vi "AlphaBeta.vi"() -> ()   [LabVIEW 2017]
uses:
  AlphaBetaAndDQ_variants/ABCtoAlphaBeta_3PhaseUnitaryMagnitude_src.vi
  AlphaBetaAndDQ_variants/AlphaBetaToABC_UnitaryMagnitude_src.vi
  AlphaBetaAndDQ_variants/ABCtoAlphaBeta_3PhasePowerInvariant_src.vi
  AlphaBetaAndDQ_variants/AlphaBetaToABC_PowerInvariant_src.vi
  AlphaBetaAndDQ_variants/ABCtoAlphaBeta_2PhaseUnitaryMagnitude_src.vi
  AlphaBetaAndDQ_variants/ABCtoAlphaBeta_2PhasePowerInvariant_src.vi
  <vilib>/Analysis/NI_AALBase.lvlib
panel:
  out "transposed array":sgl[][](graph)
  out "3 phase UM error stddev":dbl format="%0.2f"
  out "3 phase PI error stddev":dbl format="%0.2f"
  out "2 phase UM error stddev":dbl format="%0.2f"
  out "2 phase PI error stddev":dbl format="%0.2f"
  in  "Imbalance (percent)":dbl
  in  "GridImbalance":bool
  in  "Noise Magnitude (percent)":dbl
  in  "InjectAdditiveNoise":bool
  out "3 phase UM error mean":dbl format="%0.2f"
  out "3 phase UM error max":dbl
  out "3 phase PI error mean":dbl format="%0.2f"
  out "3 phase PI error max":dbl
  out "2 phase UM error mean":dbl format="%0.2f"
  out "2 phase UM error max":dbl
  in  "Magnitude":dbl=1.0
  out "2 phase PI error max":dbl
  out "2 phase PI error mean":dbl format="%0.2f"
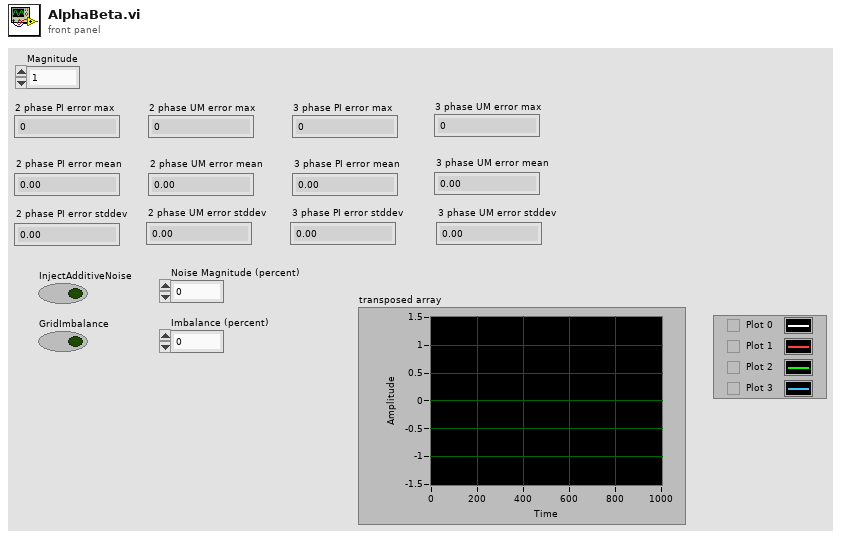
[diagram p1: front panel]
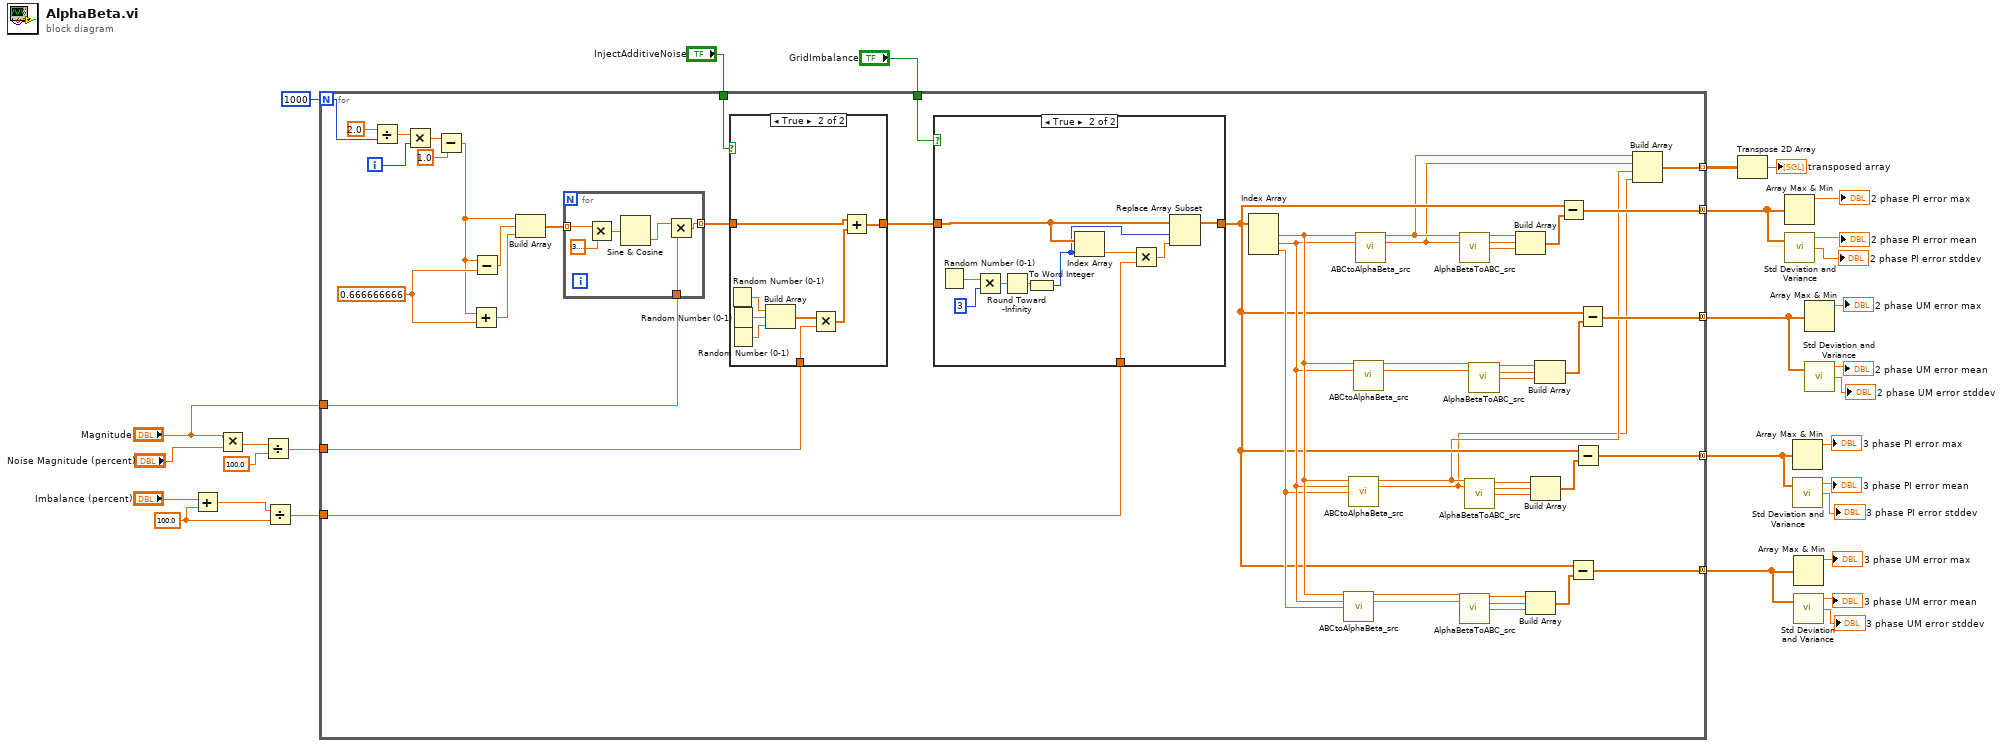
[diagram p0: block diagram]
diagram:
  w8 = 100.0 ("y")
  n1 = Add(x="Imbalance (percent)", y=w8) -> (x+y=w9:dbl)
  n2 = Multiply(x="Magnitude", y="Noise Magnitude (percent)") -> (x*y=w16:dbl)
  n3 = Divide(x=w16, y=100.0) -> (x/y=w13:dbl)
  n4 = Divide(x=w9, y=w8) -> (x/y=w7:dbl)
  n5 = for {
    N: 1000 -> [w47]
    tunnel: [w41] -> w27 mode=concatenating
    tunnel: [w40] -> w24 mode=concatenating
    tunnel: [w39] -> w21 mode=concatenating
    tunnel: [w38] -> w18 mode=concatenating
    tunnel: "Magnitude" -> [w55]
    tunnel: w13 -> [w54]
    tunnel: "InjectAdditiveNoise" -> [w53]
    tunnel: "GridImbalance" -> [w52]
    tunnel: w7 -> [w50]
    tunnel: [w31] -> w2 mode=indexing
    i -> [w45]
    w81 = 0.666666666
    n6 = Divide(x=2.0, y=w47) -> (x/y=w46:dbl)
    n7 = Multiply(x=w46, y=w45) -> (x*y=w44:dbl)
    n8 = Subtract(x=w44, y=1.0) -> (x-y=w42:dbl)
    n9 = Add(x=w42, y=w81) -> (x+y=w79:dbl)
    n10 = Subtract(x=w42, y=w81) -> (x-y=w78:dbl)
    n11 = Build Array(w42, w78, w79) -> (w80:dbl[])
    n12 = for {
      tunnel: w80 -> [w107] mode=indexing
      tunnel: [w104] -> w56 mode=indexing
      tunnel: w55 -> [w103]
      n13 = Multiply(x=w107, y=3.141592653589793) -> (x*y=w105:dbl)
      n14 = Sine & Cosine(0:w105) -> (2:w102:dbl)  [unwired: 1 out]
      n15 = Multiply(x=w102, y=w103) -> (x*y=w104:dbl)
    }
    n16 = case shown="True" w53 {
      tunnel: w56 -> [w93 w95]
      tunnel: [w93 w94] -> w51
      tunnel: w54 -> [_ w97]
      frame False {
      }
      frame True {
        n17 = Random Number (0-1)() -> (number: 0 to 1=w100:dbl)
        n18 = Random Number (0-1)() -> (number: 0 to 1=w101:dbl)
        n19 = Random Number (0-1)() -> (number: 0 to 1=w99:dbl)
        n20 = Build Array(w100, w101, w99) -> (w98:dbl[])
        n21 = Multiply(x=w98, y=w97) -> (x*y=w96:dbl[])
        n22 = Add(x=w95, y=w96) -> (x+y=w94:dbl[])
      }
    }
    n23 = case shown="True" w52 {
      tunnel: w51 -> [w82 w86]
      tunnel: w50 -> [_ w87]
      tunnel: [w82 w84] -> w49
      frame False {
      }
      frame True {
        n24 = Random Number (0-1)() -> (number: 0 to 1=w92:dbl)
        n25 = Multiply(x=w92, y=3) -> (x*y=w90:dbl)
        n26 = Round Toward -Infinity(1:w90) -> (0:w89:dbl)
        n27 = To Word Integer(number=w89) -> (16bit integer=w83:i16)
        n28 = Index Array(array=w86, index=w83) -> (element=w88:dbl)
        n29 = Multiply(x=w88, y=w87) -> (x*y=w85:dbl)
        n30 = Replace Array Subset(array=w86, new element=w85, index=w83) -> (w84:dbl[])
      }
    }
    n31 = Index Array(array=w49) -> (element #1=w59:dbl, element #2=w58:dbl, element #3=w57:dbl)  [unwired: 3 in]
    n32 = call-poly "ABCtoAlphaBeta_src.vi"("A"=w59, "B"=w58, "C"=w57) -> ("alpha"=w60:sgl, "beta"=w61:sgl)  [unwired: 11 in]
    n33 = call-poly "ABCtoAlphaBeta_src.vi"("A"=w59, "B"=w58, "C"=w57) -> ("alpha"=w33:sgl, "beta"=w32:sgl)  [unwired: 11 in]
    n34 = call-poly "ABCtoAlphaBeta_src.vi"("A"=w59, "B"=w58) -> ("alpha"=w37:sgl, "beta"=w36:sgl)  [unwired: 12 in]
    n35 = call-poly "ABCtoAlphaBeta_src.vi"("A"=w59, "B"=w58) -> ("alpha"=w35:sgl, "beta"=w34:sgl)  [unwired: 12 in]
    n36 = call-poly "AlphaBetaToABC_src.vi"("alpha"=w35, "beta"=w34) -> ("A"=w77:sgl, "B"=w76:sgl, "C"=w75:sgl)  [unwired: 11 in]
    n37 = call-poly "AlphaBetaToABC_src.vi"("alpha"=w60, "beta"=w61) -> ("A"=w63:sgl, "B"=w64:sgl, "C"=w65:sgl)  [unwired: 11 in]
    n38 = call-poly "AlphaBetaToABC_src.vi"("alpha"=w33, "beta"=w32) -> ("A"=w68:sgl, "B"=w67:sgl, "C"=w66:sgl)  [unwired: 11 in]
    n39 = call-poly "AlphaBetaToABC_src.vi"("alpha"=w37, "beta"=w36) -> ("A"=w72:sgl, "B"=w71:sgl, "C"=w70:sgl)  [unwired: 11 in]
    n40 = Build Array(w77, w76, w75) -> (w74:sgl[])
    n41 = Build Array(w63, w64, w65) -> (w62:sgl[])
    n42 = Build Array(w68, w67, w66) -> (w69:sgl[])
    n43 = Build Array(w72, w71, w70) -> (w73:sgl[])
    n44 = Subtract(x=w49, y=w74) -> (x-y=w41:dbl[])
    n45 = Subtract(x=w49, y=w62) -> (x-y=w38:dbl[])
    n46 = Subtract(x=w49, y=w69) -> (x-y=w39:dbl[])
    n47 = Subtract(x=w49, y=w73) -> (x-y=w40:dbl[])
    n48 = Build Array(w35, w34, w33, w32) -> (w31:sgl[])
  }
  n49 = Transpose 2D Array(2D array=w2) -> (transposed array=→"transposed array":sgl[][])
  n50 = Array Max & Min(array=w27) -> (max value=→"2 phase PI error max":dbl)  [unwired: 3 out]
  n51 = call <vilib>:"Std Deviation and Variance.vi"("X"=w27) -> ("mean"=→"2 phase PI error mean":dbl, "standard deviation"=→"2 phase PI error stddev":dbl)  [unwired: 1 in, 1 out]
  n52 = Array Max & Min(array=w21) -> (max value=→"3 phase PI error max":dbl)  [unwired: 3 out]
  n53 = call <vilib>:"Std Deviation and Variance.vi"("X"=w21) -> ("mean"=→"3 phase PI error mean":dbl, "standard deviation"=→"3 phase PI error stddev":dbl)  [unwired: 1 in, 1 out]
  n54 = Array Max & Min(array=w18) -> (max value=→"3 phase UM error max":dbl)  [unwired: 3 out]
  n55 = call <vilib>:"Std Deviation and Variance.vi"("X"=w18) -> ("mean"=→"3 phase UM error mean":dbl, "standard deviation"=→"3 phase UM error stddev":dbl)  [unwired: 1 in, 1 out]
  n56 = Array Max & Min(array=w24) -> (max value=→"2 phase UM error max":dbl)  [unwired: 3 out]
  n57 = call <vilib>:"Std Deviation and Variance.vi"("X"=w24) -> ("mean"=→"2 phase UM error mean":dbl, "standard deviation"=→"2 phase UM error stddev":dbl)  [unwired: 1 in, 1 out]
